vi "FPGA_HoppingScan.vi"() -> ()   [LabVIEW 2024]
uses:
  <vilib>/Platform/TimedLoop/XDataNode/timing_clust.ctl
  <vilib>/Platform/TimedLoop/XDataNode/nitl_modes.ctl
  <vilib>/Platform/TimedLoop/XDataNode/wakeup.ctl
  <vilib>/rvi/FXPMathLib/FxpDiv/subVIs/nifxpmath_Div_SimConfig.ctl
  <vilib>/rvi/Emulation/niFpgaSctlEmulationGetInTimedLoop.vi
  <vilib>/rvi/Emulation/niFpgaProcessEmulError.vi
  <vilib>/rvi/eio/common/nirviEmuTemplateMethod_errors.vi
  <vilib>/rvi/Emulation/niFpgaGetClockAttributes.vi
  <vilib>/rvi/Emulation/niFpgaEmulationReportErrorSimple.vi
  <vilib>/rvi/Emulation/niFpgaEmulationIsFPGAContextNoSignature.vi
  <vilib>/rvi/DataTransferAndStorage/Container/Common/niFpgaContainerGetUniqueNameForEmu.vi
  <vilib>/rvi/Memory/Memory_Emulation/niFpgaMemoryEmulationCacheClearOnFirstRun.vi
  <vilib>/rvi/Memory/Memory_Emulation/nirvimemoryEmulationManagerCache_MakeExclusive.vi
  <vilib>/rvi/Memory/Memory_Emulation/niFpgaMemoryEmulationValidateCache.vi
  <vilib>/rvi/Memory/Memory_Emulation/nirvimemoryEmulationManagerCache_InsertValue.vi
  <vilib>/Utility/error.llb/Clear Errors.vi
  <vilib>/rvi/Memory/Memory_Emulation/nirvimemoryEmulationManagerCache_ReleaseExclusive.vi
  <vilib>/rvi/Memory/Memory_Emulation/nirvimemoryEmulationManagerCache_GetValue.vi
  <vilib>/rvi/Memory/Memory_Emulation/nirvimemoryEmulationManagerCache_SetValue.vi
  <vilib>/rvi/FIFO/Fifo_Resource/nirvififoEmulationSetSize.vi
  <vilib>/rvi/FIFO/Fifo_Resource/nirviFifoEmulationQueueMgr.vi
  <instcachedir>/0/nirviFifoEmulationQueueMgr_E5CAEC123FF24DC58D834DCA3CDAA9B5.lvgen/nirviFifoEmulationQueueMgr_E5CAEC123FF24DC58D834DCA3CDAA9B5_001.vi
  <vilib>/rvi/errors/niFpgaSetErrorForExecOnDevCompSimple.vi
  <vilib>/rvi/eio/common/nirviEmuReportErrorAndStop.vi
  <vilib>/rvi/FIFO/Fifo_Resource/nirvififoEmulationCreateLock.vi
  <vilib>/rvi/FIFO/Fifo_Resource/nirvififoEmulationObtainLock.vi
  <vilib>/rvi/FIFO/Fifo_Resource/nirvififoEmulationReleaseLock.vi
  <vilib>/rvi/occurrence/nirviWaitOnOccurrenceBase.vi
  <vilib>/rvi/errors/nirviReportUnexpectedCaseInternalError.vi
  <vilib>/rvi/errors/nirviReportUnexpectedCaseInternalError (U32).vi
  <vilib>/rvi/Emulation/niFpgaCriticalErrorInLSC.vi
  <vilib>/rvi/Memory/Memory_Emulation/nirvimemoryFastEmulation.vi
  <vilib>/rvi/Memory/Memory_Emulation/nirvimemoryEmulation.vi
  <vilib>/eio/utilities/niEioResolveVilibRelativePath.vi
  <vilib>/rvi/interface/RandomDataEmulation/niFpgaRandomDataHandleErrors.vi
  <vilib>/rvi/FXPMathLib/FxpDiv/simVIs/DllFxpDivTemp_sub.vi
  <vilib>/rvi/FIFO/Fifo_Resource/nirvififoEmulationDetermineInputValidOut.vi
  <vilib>/eio/EIONode/EIONode.xnode
  <vilib>/rvi/DataTransferAndStorage/Container/XNode/niFpgaContainer.xnode
  <vilib>/rvi/DataTransferAndStorage/Register/Emulation/niFpgaRegisterEmulation.vi
  <vilib>/rvi/FIFO/Fifo_Resource/nirvififoEmulationGetNumberOfElementsToRead.vi
  <vilib>/rvi/FIFO/Fifo_Resource/nirvififoEmulationRead.vi
  <vilib>/platform/TimedLoop/XDataNode/XDataNode.xnode
  <vilib>/rvi/interface/RandomDataEmulation/nirviRandomDataFpgaReadWriteTemplate.vi
  <vilib>/rvi/FXPMathLib/FxpSub/XNode/nifxpmath_Sub.xnode
  <vilib>/rvi/FXPMathLib/FxpAdd/XNode/nifxpmath_Add.xnode
  <vilib>/rvi/FXPMathLib/FxpMul/XNode/nifxpmath_Multiplier.xnode
  <vilib>/rvi/FXPMathLib/FxpDiv/XNode/nifxpmath_Div.xnode
  <vilib>/rvi/FIFO/Fifo_Resource/nirvififoEmulationWrite.vi
  <vilib>/rvi/FXPMathLib/sim/FxpSim.dll
  <vilib>/Platform/TimedLoop/XDataNode/XDNodeRunTimeDep.lvlib
panel:
  in  "DelayPoints":i32
  in  "Halting Threshold":fxp<+/-,48,16>
  out "point_scanned":u32
  in  "TotalPoints":u32
  in  "RetRate us":i32
  in  "AppRate_NF us":i32
  in  "AppRate_FF us":i32
  in  "Recording Threshold":fxp<+/-,48,16>
  in  "stop":bool
  out "TargetDone?":bool
  out "ScanFinished?":bool
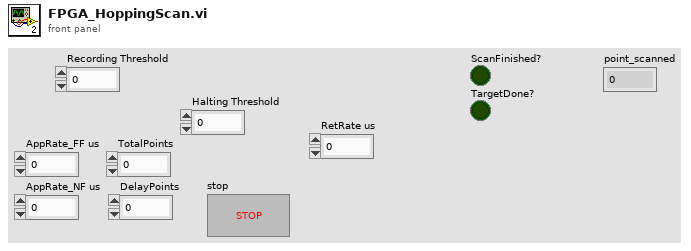
[diagram p1: front panel]
types:
  T1 = typedef "XDNodeRunTimeDep.lvlib/timing_clust.ctl" = cluster{"Expected End [f-1]":u64, "Actual End [f-1]":u64, "Finished Late? [f-1]":bool, "Expected End [i-1]":u64, "Actual End [i-1]":u64, "Finished Late? [i-1]":bool, "Expected Start [i]":u64, "Actual Start [i]":u64, "Expected Start [f]":u64, "Actual Start [f]":u64, "Source Name":string, "Structure Name":string, "Period":i64, "Deadline":i64, "Offset":i64, "Start":i64, "Priority":i32, "Timeout":i32, "Mode":T2, "Wakeup Reason":T3, "Error":errorcluster, "Source Type":string, "Secondary Source Type":string, "Global End Time":u64, "Global Start Time":u64, "Frame Duration":u64, "Iteration Duration":u64, "Assigned CPU":i32, "I/O Scan Engine Mode":u32}
  T2 = typedef "XDNodeRunTimeDep.lvlib/nitl_modes.ctl" = enum32{"No Change", "Process missed periods, maintain original phase", "Discard missed periods, maintain original phase", "Process missed periods, ignore original phase", "Discard missed periods, ignore original phase"}
  T3 = typedef "XDNodeRunTimeDep.lvlib/wakeup.ctl" = enum32{"Normal", "Aborted", "Asynchronous wakeup", "Timing source error", "Timed loop error", "Timeout"}
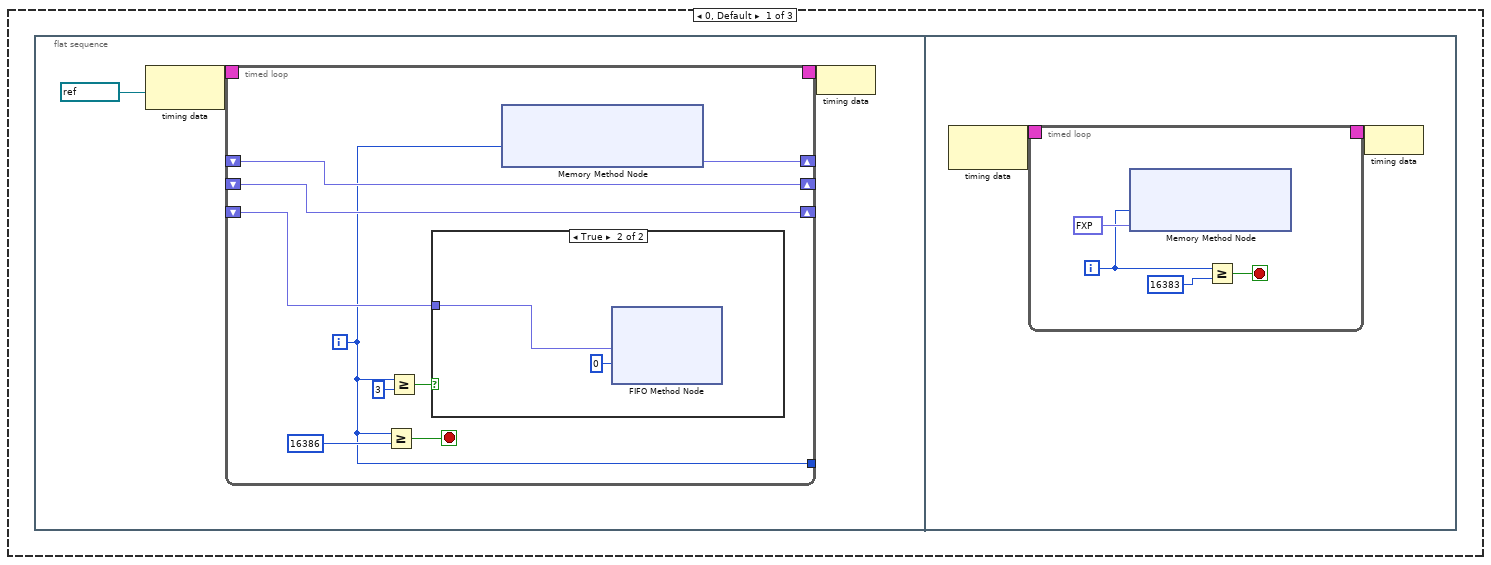
[diagram p3: hidden frame]
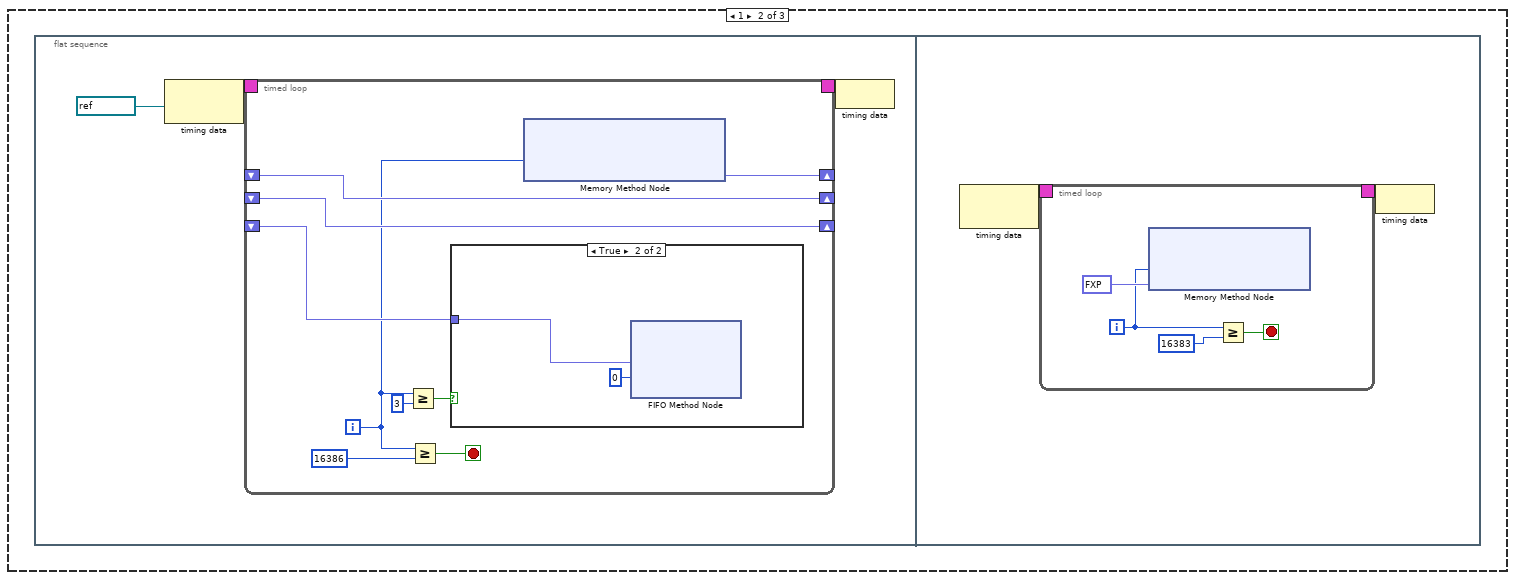
[diagram p5: hidden frame]
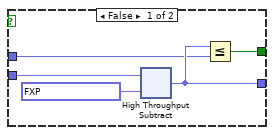
[diagram p13: hidden frame]
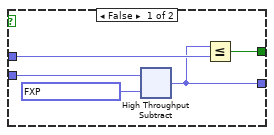
[diagram p14: hidden frame]
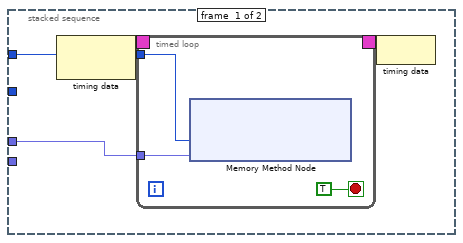
[diagram p16: hidden frame]
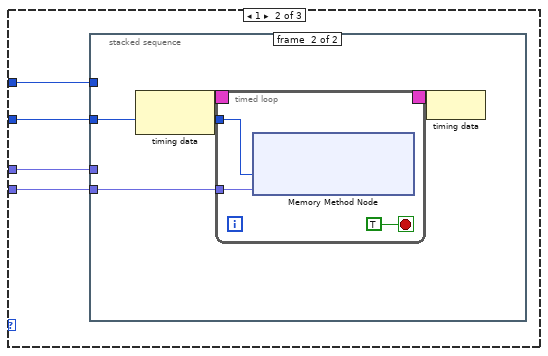
[diagram p17: hidden frame]
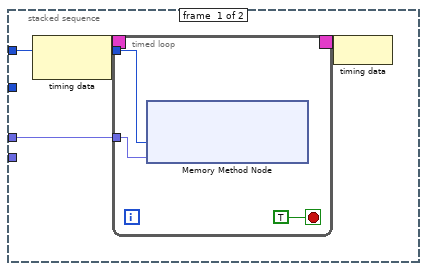
[diagram p18: hidden frame]
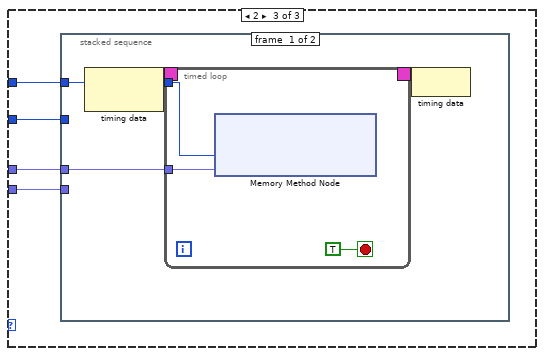
[diagram p19: hidden frame]
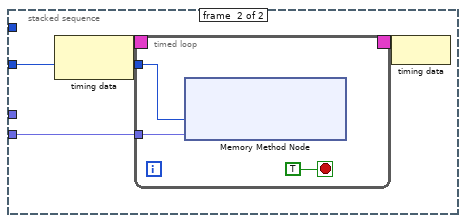
[diagram p20: hidden frame]
diagram:
  n1 = flat-sequence {
    tunnel: [w5] -> w1
    tunnel: w1 -> [w18]
    frame #0 {
      w4 = fxp<+/-,20,5> 0.0 ("Connector0/AO0")
      n2 = xnode "FPGA I/O Node"("Connector0/AO0"=w4, "Connector0/AO1"=w4, "Connector0/AO2"=w4) -> ()  [unwired: 3 in, 3 out]
      "ScanFinished?" <- FALSE
      "TargetDone?" <- FALSE
    }
    frame #1 {
      n3 = Generate Occurrence() -> (w5:refnum<k4>)
      n4 = call "Wait"("Count(mSec)"=u8 200) -> ()  [unwired: 1 out]
    }
    frame #2 {
      n5 = while {
        tunnel: w18 -> [w135]
        stop <- w137 stop-if-true
        n6 = xnode ("Register Read")() -> ("Data"=w138:bool)  [unwired: 1 in, 1 out]
        n7 = xnode ("FIFO Method Node")() -> ("Number of Elements to Read"=w141:u32)  [unwired: 1 in, 1 out]
        n8 = local read "ScanFinished?"() -> (w136:bool)
        n9 = Or(x=w138, y=w136) -> (x .or. y?=w137:bool)
        n10 = Greater Or Equal?(x=w141, y=u32 6) -> (x >= y?=w139:bool)
        n11 = case shown="True" w139 {
          tunnel: w135 -> [_ w142]
          frame False {
          }
          frame True {
            n12 = First Call?() -> (First Call?: T/F=w143:bool)
            n13 = case shown="True" w143 {
              tunnel: w142 -> [_ w144]
              frame False {
              }
              frame True {
                n14 = flat-sequence {
                  tunnel: [w147] -> w145
                  tunnel: w144 -> [w147]
                  tunnel: w145 -> [w148]
                  frame #0 {
                    n15 = call "Wait3"("Count(mSec)"=u8 4) -> ()  [unwired: 1 out]
                  }
                  frame #1 {
                    n16 = Set Occurrence(w148) -> ()
                  }
                }
              }
            }
          }
        }
      }
      n17 = while {
        tunnel: w18 -> [w120]
        stop <- w117 stop-if-true
        n18 = flat-sequence {
          tunnel: ["stop"] -> w122
          tunnel: w120 -> [w124]
          tunnel: [w124] -> w118
          tunnel: w122 -> [w127]
          tunnel: [w127] -> w121
          tunnel: [w126] -> w119
          tunnel: w118 -> [w126]
          tunnel: w121 -> [w131]
          tunnel: w119 -> [w130]
          tunnel: [w129] -> w117
          frame #0 {
            n19 = case shown="True" "stop" {
              tunnel: "stop" -> [_ w125]
              frame False {
              }
              frame True {
                n20 = xnode ("Register Write")("Data"=w125) -> ()  [unwired: 1 in, 1 out]
              }
            }
          }
          frame #1 {
            n21 = call "Wait2"("Count(uSec)"=u8 200) -> ()  [unwired: 1 out]
          }
          frame #2 {
            n22 = xnode ("Register Read")() -> ("Data"=w132:bool)  [unwired: 1 in, 1 out]
            n23 = local read "ScanFinished?"() -> (w133:bool)
            n24 = Compound Arithmetic op=OR(w133, w132, w131) -> (w129:bool)
            n25 = case shown="True" w129 {
              tunnel: w130 -> [_ w134]
              frame False {
              }
              frame True {
                n26 = Set Occurrence(w134) -> ()
              }
            }
          }
        }
      }
      n27 = flat-sequence {
        tunnel: w18 -> [w149]
        tunnel: [fxp<+/-,48,16> 0.0 ("Threshold")] -> w17
        tunnel: [w151] -> w15
        tunnel: [u8 0] -> w12
        tunnel: w17 -> [w154]
        tunnel: [w155] -> w16
        tunnel: w15 -> [w155]
        tunnel: [w154] -> w14
        tunnel: [w153] -> w13
        tunnel: w12 -> [w153]
        tunnel: w16 -> [w160]
        tunnel: w14 -> [w159]
        tunnel: w13 -> [w158]
        tunnel: [w157] -> w11
        tunnel: w11 -> [w1114]
        tunnel: [w1112] -> w10
        tunnel: [w1111] -> w8
        tunnel: w10 -> [w1126]
        tunnel: [w1126] -> w9
        tunnel: w8 -> [w1125]
        tunnel: [w1125] -> w7
        tunnel: w9 -> [w1130]
        tunnel: w7 -> [w1127]
        frame #0 {
          n28 = Wait on Occurrence(2:w149) -> ()  [unwired: 2 in, 1 out]
        }
        frame #1 {
          # "z piezo voltage"
          # "Swapchain indicator"
          n29 = xnode ("Register Read")() -> ("Data"=w151:bool)  [unwired: 1 in, 1 out]
        }
        frame #2 {
          n30 = call "Wait4"("Count(mSec)"=u8 4) -> ()  [unwired: 1 out]
        }
        frame #3 {
          n31 = case shown="False" w160 {
            tunnel: w159 -> [w163 w1110]
            tunnel: w158 -> [w162 _]
            tunnel: [w161 w1110] -> w157
            frame False {
              n32 = while {
                shift-right: [w171] -> w161
                shift-left: w163 -> [w205]
                shift-right: [w170] -> _
                shift-left: w162 -> [w184]
                stop <- w169 stop-if-true
                n33 = flat-sequence {
                  tunnel: w205 -> [w207]
                  tunnel: [w209] -> w204
                  tunnel: [w208] -> w200
                  tunnel: [w207] -> w189
                  tunnel: w184 -> [w206]
                  tunnel: [w206] -> w183
                  tunnel: w204 -> [w217]
                  tunnel: [w217] -> w203
                  tunnel: w200 -> [w216]
                  tunnel: [w216] -> w199
                  tunnel: w189 -> [w215]
                  tunnel: [w215] -> w188
                  tunnel: w183 -> [w214]
                  tunnel: [w214] -> w182
                  tunnel: w203 -> [w244]
                  tunnel: [w244] -> w202
                  tunnel: [w237] -> w201
                  tunnel: w199 -> [w243]
                  tunnel: [w243] -> w198
                  tunnel: [w238] -> w196
                  tunnel: [w241] -> w194
                  tunnel: [w240] -> w193
                  tunnel: [w239] -> w192
                  tunnel: w188 -> [w236]
                  tunnel: w182 -> [w242]
                  tunnel: [w242] -> w181
                  tunnel: [w233] -> w168
                  tunnel: [w235] -> w164
                  tunnel: w202 -> [w280]
                  tunnel: w201 -> [w281]
                  tunnel: w198 -> [w279]
                  tunnel: [w279] -> w197
                  tunnel: w196 -> [w278]
                  tunnel: [w278] -> w195
                  tunnel: w194 -> [w277]
                  tunnel: w193 -> [w275]
                  tunnel: w192 -> [w274]
                  tunnel: [w277] -> w191
                  tunnel: [w272] -> w187
                  tunnel: w181 -> [w276]
                  tunnel: [w276] -> w180
                  tunnel: [w275] -> w177
                  tunnel: [w274] -> w176
                  tunnel: w168 -> [w273]
                  tunnel: [w273] -> w167
                  tunnel: w164 -> [w272]
                  tunnel: w197 -> [w308]
                  tunnel: w195 -> [w309]
                  tunnel: w191 -> [w307]
                  tunnel: [w307] -> w190
                  tunnel: w187 -> [w306]
                  tunnel: [w306] -> w186
                  tunnel: w180 -> [w305]
                  tunnel: [w305] -> w178
                  tunnel: w177 -> [w304]
                  tunnel: w176 -> [w303]
                  tunnel: [w304] -> w175
                  tunnel: [w303] -> w174
                  tunnel: w167 -> [w302]
                  tunnel: [w302] -> w166
                  tunnel: w190 -> [w335]
                  tunnel: w186 -> [w334]
                  tunnel: [w334] -> w185
                  tunnel: [w333] -> w179
                  tunnel: w178 -> [w333]
                  tunnel: w175 -> [w332]
                  tunnel: w174 -> [w331]
                  tunnel: [w332] -> w173
                  tunnel: [w331] -> w172
                  tunnel: w166 -> [w330]
                  tunnel: [w330] -> w165
                  tunnel: w185 -> [w350]
                  tunnel: w179 -> [w349]
                  tunnel: w173 -> [w348]
                  tunnel: w172 -> [w347]
                  tunnel: [w346] -> w170
                  tunnel: [w345] -> w171
                  tunnel: [w344] -> w169
                  tunnel: w165 -> [w340]
                  frame #0 {
                    # "Data from target to host:\n0, 1: X, Y piezo voltage\n2, 3: X, Y piezo idx\n4: Z piezo voltage\n5: baseline current\n(6-8105): Z voltage\n(8106-16205): current"
                    # "Data from host to target:\n0, 1: X, Y piezo voltage\n2, 3: X, Y piezo idx\n4: distance (piezo voltage) to the last point\n5: retract height, \nall negative cases won't trigger approach of z piezo\nif -20, keep z and move xy\nif -30, full retract for z and move xy"
                    n34 = for {
                      N: 2 -> [_]
                      shift-right: [w213] -> w208
                      shift-left: _ -> [w211]
                      shift-right: [w211] -> w209
                      shift-left: _ -> [_]
                      i -> [w212]
                      n35 = xnode ("Memory Method Node")("Address"=w212) -> ("Data"=w213:fxp<+/-,48,16>)  [unwired: 1 in, 1 out]
                    }
                  }
                  frame #1 {
                    # "y"
                    # "x"
                    n36 = while {
                      shift-right: [w221] -> _
                      shift-left: i16 0 -> [w220]
                      stop <- w222 stop-if-true
                      n37 = xnode ("FIFO Method Node")("Timeout"=8192) -> ("Element"=w219:fxp<+/-,48,16>, "Timed Out?"=w226:bool)  [unwired: 1 in, 1 out]
                      n38 = Increment(x=w220) -> (x+1=w229:i16)
                      n39 = xnode ("Register Read")() -> ("Data"=w223:bool)  [unwired: 1 in, 1 out]
                      n40 = Select(t=w220, s=w226, f=w229) -> (s? t:f=w221:i16)
                      n41 = Not(x=w226) -> (.not. x?=w225:bool)
                      n42 = Equal?(x=w220, y=i16 5) -> (x = y?=w227:bool)
                      n43 = And(x=w227, y=w225) -> (x .and. y?=w224:bool)
                      n44 = xnode ("Memory Method Node")("Address"=w220, "Data"=w219) -> ()  [unwired: 1 in, 1 out]
                      n45 = Or(x=w224, y=w223) -> (x .or. y?=w222:bool)
                    }
                  }
                  frame #2 {
                    # "0"
                    # "5"
                    n46 = for {
                      N: 6 -> [_]
                      shift-right: [w270] -> w233
                      shift-left: _ -> [w269]
                      shift-right: [w269] -> w241
                      shift-left: _ -> [w268]
                      shift-right: [w268] -> w240
                      shift-left: _ -> [w267]
                      shift-right: [w267] -> w239
                      shift-left: _ -> [w266]
                      shift-right: [w266] -> w238
                      shift-left: _ -> [w265]
                      shift-right: [w265] -> w237
                      shift-left: _ -> [_]
                      i -> [w271]
                      n47 = xnode ("Memory Method Node")("Address"=w271) -> ("Data"=w270:fxp<+/-,48,16>)  [unwired: 1 in, 1 out]
                    }
                    n48 = Equal?(x=w233, y=fxp<+/-,48,16> -30.0) -> (x = y?=w232:bool)
                    n49 = case shown="True" w232 {
                      tunnel: w236 -> [w246 w250]
                      tunnel: [w246 w249] -> w235
                      tunnel: fxp<+/-,48,16> 0.0048828125 ("y") -> [_ w248]
                      frame False {
                      }
                      frame True {
                        n50 = flat-sequence {
                          tunnel: w250 -> [w253]
                          tunnel: w248 -> [w251]
                          tunnel: [w252] -> w247
                          tunnel: [w264] -> w249
                          tunnel: w247 -> [w264]
                          frame #0 {
                            n51 = while {
                              shift-right: [w257] -> w252
                              shift-left: w253 -> [w262]
                              tunnel: w251 -> [w256]
                              stop <- w258 stop-if-true
                              w259 = fxp<+/-,48,16> 0.0 ("y")
                              n52 = xnode "High Throughput Subtract"("x"=w262, "y"=w256) -> ("x-y"=w260:fxp<+/-,48,16>)
                              n53 = xnode ("Register Read")() -> ("Data"=w261:bool)  [unwired: 1 in, 1 out]
                              n54 = Less Or Equal?(x=w260, y=w259) -> (x <= y?=w254:bool)
                              n55 = Select(t=w259, s=w254, f=w260) -> (s? t:f=w257:fxp<+/-,48,16>)
                              n56 = local read "RetRate us"() -> (w255:i32)
                              n57 = xnode "FPGA I/O Node"("Connector0/AO2"=w257) -> ()  [unwired: 1 in, 1 out]
                              n58 = Compound Arithmetic op=OR(w254, w261) -> (w258:bool)
                              n59 = call "Wait10"("Count(uSec)"=w255) -> ()  [unwired: 1 out]
                            }
                          }
                          frame #1 {
                            n60 = call "Wait17"("Count(mSec)"=u16 2 ("Count(uSec)")) -> ()  [unwired: 1 out]
                          }
                        }
                      }
                    }
                  }
                  frame #3 {
                    n61 = xnode "High Throughput Subtract"("x"=w280, "y"=w281) -> ("x-y"=w283:fxp<+/-,48,16>)
                    n62 = Less Or Equal To 0?(x=w283) -> (x <= 0?=w282:bool)
                    n63 = while {
                      tunnel: w282 -> [w291]
                      tunnel: w281 -> [w290]
                      shift-right: [w284] -> _
                      shift-left: w280 -> [w286]
                      stop <- w287 stop-if-true
                      n64 = case shown="True" w291 {
                        tunnel: w290 -> [w292 w297]
                        tunnel: w286 -> [w295 w301]
                        tunnel: [w294 w299] -> w285
                        tunnel: [w293 w298] -> w284
                        frame False {
                          n65 = xnode "High Throughput Subtract"("x"=w295, "y"=fxp<+/-,48,16> 0.00030517578125) -> ("x-y"=w293:fxp<+/-,48,16>)
                          n66 = Less Or Equal?(x=w293, y=w292) -> (x <= y?=w294:bool)
                        }
                        frame True {
                          n67 = xnode ("High Throughput Add")("x"=w301, "y"=fxp<+/-,48,16> 0.00030517578125) -> ("x+y"=w298:fxp<+/-,48,16>)
                          n68 = Greater Or Equal?(x=w298, y=w297) -> (x >= y?=w299:bool)
                        }
                      }
                      n69 = call "Wait5"("Count(uSec)"=u32 70) -> ()  [unwired: 1 out]
                      n70 = xnode ("Register Read")() -> ("Data"=w288:bool)  [unwired: 1 in, 1 out]
                      n71 = xnode "FPGA I/O Node"("Connector0/AO0"=w284) -> ()  [unwired: 1 in, 1 out]
                      n72 = Or(x=w285, y=w288) -> (x .or. y?=w287:bool)
                    }
                  }
                  frame #4 {
                    n73 = xnode "High Throughput Subtract"("x"=w308, "y"=w309) -> ("x-y"=w311:fxp<+/-,48,16>)
                    n74 = Less Or Equal To 0?(x=w311) -> (x <= 0?=w310:bool)
                    n75 = while {
                      tunnel: w310 -> [w319]
                      tunnel: w309 -> [w318]
                      shift-right: [w312] -> _
                      shift-left: w308 -> [w314]
                      stop <- w315 stop-if-true
                      n76 = case shown="True" w319 {
                        tunnel: w318 -> [w321 w326]
                        tunnel: w314 -> [w323 w329]
                        tunnel: [w322 w327] -> w313
                        tunnel: [w320 w325] -> w312
                        frame False {
                          n77 = xnode "High Throughput Subtract"("x"=w323, "y"=fxp<+/-,48,16> 0.00030517578125) -> ("x-y"=w320:fxp<+/-,48,16>)
                          n78 = Less Or Equal?(x=w320, y=w321) -> (x <= y?=w322:bool)
                        }
                        frame True {
                          n79 = xnode ("High Throughput Add")("x"=w329, "y"=fxp<+/-,48,16> 0.00030517578125) -> ("x+y"=w325:fxp<+/-,48,16>)
                          n80 = Greater Or Equal?(x=w325, y=w326) -> (x >= y?=w327:bool)
                        }
                      }
                      n81 = call "Wait6"("Count(uSec)"=u32 70) -> ()  [unwired: 1 out]
                      n82 = xnode ("Register Read")() -> ("Data"=w316:bool)  [unwired: 1 in, 1 out]
                      n83 = xnode "FPGA I/O Node"("Connector0/AO1"=w312) -> ()  [unwired: 1 in, 1 out]
                      n84 = Or(x=w313, y=w316) -> (x .or. y?=w315:bool)
                    }
                  }
                  frame #5 {
                    n85 = xnode ("High Throughput Multiply")("x"=w335, "y"=fxp<+/-,48,16> 1600.0) -> ("x*y"=w337:fxp<+/-,52,20>)
                    n86 = To Unsigned Long Integer(number=w337) -> (unsigned 32bit integer=w338:u32)
                    n87 = call "Wait7"("Count(uSec)"=w338) -> ()  [unwired: 1 out]
                  }
                  frame #6 {
                    # "Y, X idx"
                    n88 = xnode ("Register Read")() -> ("Data"=w343:bool)  [unwired: 1 in, 1 out]
                    n89 = Less Or Equal?(x=w340, y=fxp<+/-,48,16> -20.0) -> (x <= y?=w341:bool)
                    n90 = Or(x=w341, y=w343) -> (x .or. y?=w342:bool)
                    n91 = case shown="False" w342 {
                      tunnel: w350 -> [w370 w1109]
                      tunnel: w349 -> [w368 w1108]
                      tunnel: w348 -> [w362 _]
                      tunnel: w347 -> [w361 _]
                      tunnel: [w359 w1109] -> w345
                      tunnel: [w360 w1108] -> w346
                      tunnel: [w358 w1105] -> w344
                      tunnel: w341 -> [_ w1107]
                      tunnel: w340 -> [w354 _]
                      frame False {
                        n92 = flat-sequence {
                          tunnel: [w376] -> w373
                          tunnel: [w381] -> w372
                          tunnel: [w380] -> w371
                          tunnel: w370 -> [w379]
                          tunnel: [w379] -> w369
                          tunnel: w368 -> [w378]
                          tunnel: [w378] -> w367
                          tunnel: [0] -> w366
                          tunnel: [w376] -> w353
                          tunnel: [FALSE] -> w351
                          tunnel: w373 -> [w427]
                          tunnel: w372 -> [w426]
                          tunnel: w371 -> [w425]
                          tunnel: w369 -> [w424]
                          tunnel: w367 -> [w423]
                          tunnel: w366 -> [w418]
                          tunnel: [w422] -> w365
                          tunnel: [w421] -> w364
                          tunnel: [w420] -> w363
                          tunnel: w353 -> [w419]
                          tunnel: [w419] -> w352
                          tunnel: w351 -> [w417]
                          tunnel: w365 -> [w759]
                          tunnel: w364 -> [w761]
                          tunnel: w363 -> [w762]
                          tunnel: w362 -> [w764]
                          tunnel: w361 -> [w763]
                          tunnel: [w760] -> w357
                          tunnel: [w759] -> w356
                          tunnel: [w756] -> w355
                          tunnel: w352 -> [w755]
                          tunnel: [w1085] -> w358
                          tunnel: [w1084] -> w359
                          tunnel: [w1086] -> w360
                          tunnel: w357 -> [w1086]
                          tunnel: w356 -> [w1081]
                          tunnel: w355 -> [w1085]
                          tunnel: w354 -> [w1082]
                          frame #0 {
                            n93 = for {
                              N: 64 -> [_]
                              shift-right: [w414] -> w384
                              shift-left: fxp<+/-,48,16> 0.0 -> [w415]
                              n94 = xnode "FPGA I/O Node"() -> ("Connector0/AI3"=w416:fxp<+/-,27,5>)  [unwired: 1 in, 1 out]
                              n95 = xnode ("High Throughput Add")("x"=w416, "y"=w415) -> ("x+y"=w414:fxp<+/-,48,16>)
                            }
                            n96 = local read "Halting Threshold"() -> (w375:fxp<+/-,48,16>)
                            n97 = local read "Recording Threshold"() -> (w382:fxp<+/-,48,16>)
                            n98 = xnode "High Throughput Divide"("x"=w384, "y"=fxp<+/-,48,16> 64.0) -> ("x/y"=w376:fxp<+/-,48,16>)
                            n99 = xnode ("High Throughput Multiply")("x"=w376, "y"=w382) -> ("x*y"=w381:fxp<+/-,48,16>)
                            n100 = xnode ("High Throughput Multiply")("x"=w376, "y"=w375) -> ("x*y"=w380:fxp<+/-,48,16>)
                          }
                          frame #1 {
                            n101 = while {
                              tunnel: w427 -> [w492]
                              tunnel: w426 -> [w491]
                              tunnel: w425 -> [w490]
                              shift-right: [w469] -> w422
                              shift-left: w424 -> [w489]
                              shift-right: [w468] -> w421
                              shift-left: w423 -> [w488]
                              shift-right: [w449] -> _
                              shift-left: w418 -> [w487]
                              shift-right: [w450] -> _
                              shift-left: w418 -> [w476]
                              tunnel: [w460] -> w420
                              shift-right: [w434] -> _
                              shift-left: w418 -> [w438]
                              shift-right: [w428] -> _
                              shift-left: w417 -> [w432]
                              stop <- w465 stop-if-true
                              n102 = flat-sequence {
                                tunnel: w476 -> [w496]
                                tunnel: w487 -> [w497]
                                tunnel: w488 -> [w498]
                                tunnel: w489 -> [w499]
                                tunnel: w490 -> [w500]
                                tunnel: w491 -> [w501]
                                tunnel: w492 -> [w502]
                                tunnel: [w502] -> w459
                                tunnel: [w501] -> w458
                                tunnel: [w500] -> w457
                                tunnel: [w499] -> w456
                                tunnel: [w498] -> w455
                                tunnel: [w497] -> w454
                                tunnel: [w496] -> w453
                                tunnel: [w495] -> w452
                                tunnel: [w494] -> w439
                                tunnel: w438 -> [w494]
                                tunnel: [w493] -> w433
                                tunnel: w432 -> [w493]
                                tunnel: [w550] -> w486
                                tunnel: [w546] -> w485
                                tunnel: [w545] -> w484
                                tunnel: [w533] -> w480
                                tunnel: [w530] -> w479
                                tunnel: [w544] -> w475
                                tunnel: [w543] -> w473
                                tunnel: [w542] -> w470
                                tunnel: [w523] -> w467
                                tunnel: [w504] -> w463
                                tunnel: [w535] -> w461
                                tunnel: w459 -> [w557]
                                tunnel: w458 -> [w555]
                                tunnel: w457 -> [w525]
                                tunnel: w456 -> [w547]
                                tunnel: w455 -> [w543]
                                tunnel: w454 -> [w520]
                                tunnel: w453 -> [w544]
                                tunnel: w452 -> [w529]
                                tunnel: [w529] -> w451
                                tunnel: w439 -> [w509]
                                tunnel: [w510] -> w436
                                tunnel: w433 -> [w506]
                                tunnel: [w504] -> w431
                                tunnel: w486 -> [w630]
                                tunnel: w485 -> [w629]
                                tunnel: w484 -> [w631]
                                tunnel: [w631] -> w483
                                tunnel: [w630] -> w482
                                tunnel: [w629] -> w481
                                tunnel: w480 -> [w628]
                                tunnel: w479 -> [w627]
                                tunnel: [w628] -> w478
                                tunnel: [w627] -> w477
                                tunnel: w475 -> [w626]
                                tunnel: [w626] -> w474
                                tunnel: w473 -> [w625]
                                tunnel: [w625] -> w472
                                tunnel: [w624] -> w471
                                tunnel: w470 -> [w624]
                                tunnel: w467 -> [w623]
                                tunnel: [w623] -> w466
                                tunnel: [w622] -> w464
                                tunnel: w463 -> [w622]
                                tunnel: [w621] -> w462
                                tunnel: w461 -> [w621]
                                tunnel: w451 -> [w620]
                                tunnel: [w620] -> w442
                                tunnel: [w619] -> w437
                                tunnel: w436 -> [w619]
                                tunnel: w431 -> [w618]
                                tunnel: [w618] -> w430
                                tunnel: w483 -> [w638]
                                tunnel: w482 -> [w652]
                                tunnel: w481 -> [w643]
                                tunnel: w478 -> [w645]
                                tunnel: w477 -> [w644]
                                tunnel: w474 -> [w646]
                                tunnel: w472 -> [w642]
                                tunnel: w471 -> [w648]
                                tunnel: w466 -> [w641]
                                tunnel: w464 -> [w640]
                                tunnel: w462 -> [w639]
                                tunnel: [w652] -> w448
                                tunnel: [w647] -> w447
                                tunnel: [w643] -> w446
                                tunnel: [w642] -> w445
                                tunnel: [w641] -> w444
                                tunnel: [w639] -> w443
                                tunnel: w442 -> [w636]
                                tunnel: [w636] -> w441
                                tunnel: [w635] -> w440
                                tunnel: w437 -> [w633]
                                tunnel: [w633] -> w435
                                tunnel: w430 -> [w632]
                                tunnel: [w632] -> w429
                                tunnel: [w749] -> w460
                                tunnel: [w750] -> w465
                                tunnel: [w751] -> w468
                                tunnel: [w752] -> w469
                                tunnel: [w753] -> w450
                                tunnel: [w754] -> w449
                                tunnel: w448 -> [w754]
                                tunnel: w447 -> [w753]
                                tunnel: w446 -> [w752]
                                tunnel: w445 -> [w751]
                                tunnel: w444 -> [w750]
                                tunnel: w443 -> [w749]
                                tunnel: w441 -> [w747]
                                tunnel: w440 -> [w746]
                                tunnel: [w740] -> w434
                                tunnel: w435 -> [w740]
                                tunnel: w429 -> [w739]
                                tunnel: [w739] -> w428
                                frame #0 {
                                n103 = call "Tick Count"() -> ("Tick Count(uSec)"=w495:u32)
                                }
                                frame #1 {
                                w507 = 16
                                w522 = 1 ("y")
                                w548 = fxp<+/-,48,16> 0.0 ("y")
                                # "brake zone"
                                # "recording zone"
                                # "speed switch"
                                n104 = for {
                                N: w507 -> [_]
                                shift-right: [w615] -> w534
                                shift-left: w548 -> [w616]
                                shift-right: [w612] -> w532
                                shift-left: w548 -> [w614]
                                n105 = xnode "FPGA I/O Node"() -> ("Connector0/AI2"=w617:fxp<+/-,27,5>, "Connector0/AI3"=w613:fxp<+/-,27,5>)  [unwired: 2 in, 2 out]
                                n106 = xnode ("High Throughput Add")("x"=w614, "y"=w613) -> ("x+y"=w612:fxp<+/-,48,16>)
                                n107 = xnode ("High Throughput Add")("x"=w617, "y"=w616) -> ("x+y"=w615:fxp<+/-,48,16>)
                                }
                                n108 = To Fixed-Point(number=w507) -> (fixed-point=w531:fxp<+/-,48,16>)  [unwired: 1 in]
                                n109 = local read "DelayPoints"() -> (w503:i32)
                                n110 = Not Equal To 0?(x=w509) -> (x != 0?=w508:bool)
                                n111 = Greater Or Equal?(x=w509, y=w503) -> (x >= y?=w516:bool)
                                n112 = Select(t=fxp<+/-,48,16> 0.0 ("y"), s=w508, f=fxp<+/-,48,16> 0.00030517578125 ("y")) -> (s? t:f=w517:fxp<+/-,48,16>)
                                n113 = xnode "High Throughput Divide"("x"=w534, "y"=w531) -> ("x/y"=w533:fxp<+/-,48,16>)
                                n114 = xnode "High Throughput Divide"("x"=w532, "y"=w531) -> ("x/y"=w530:fxp<+/-,48,16>)
                                n115 = xnode ("High Throughput Add")("x"=w517, "y"=w547) -> ("x+y"=w536:fxp<+/-,48,16>)
                                n116 = xnode "High Throughput Subtract"("x"=w557, "y"=w530) -> ("x-y"=w556:fxp<+/-,48,16>)
                                n117 = Absolute Value(x=w556) -> (abs(x)=w526:fxp<+,48,16>)
                                n118 = Less Or Equal?(x=w536, y=fxp<+/-,48,16> 9.75) -> (x <= y?=w538:bool)
                                n119 = Greater Or Equal?(x=w536, y=fxp<+/-,48,16> -0.125) -> (x >= y?=w539:bool)
                                n120 = And(x=w539, y=w538) -> (x .and. y?=w537:bool)
                                n121 = Greater Or Equal?(x=w526, y=w555) -> (x >= y?=w554:bool)
                                n122 = Less Or Equal?(x=w526, y=w525) -> (x <= y?=w528:bool)
                                n123 = Increment(x=w520) -> (x+1=w553:i32)
                                n124 = Select(t=w553, s=w554, f=0) -> (s? t:f=w550:i32)
                                n125 = xnode ("Register Read")() -> ("Data"=w542:bool)  [unwired: 1 in, 1 out]
                                n126 = Greater Or Equal?(x=w550, y=w522) -> (x >= y?=w505:bool)
                                n127 = Equal?(x=w550, y=0 ("f")) -> (x = y?=w549:bool)
                                n128 = Not(x=w528) -> (.not. x?=w535:bool)
                                n129 = Or(x=w506, y=w505) -> (x .or. y?=w504:bool)
                                n130 = Select(t=1 ("y"), s=w504, f=0) -> (s? t:f=w512:i32)
                                n131 = Add(x=w509, y=w512) -> (x+y=w511:i32)
                                n132 = Select(t=0, s=w516, f=w511) -> (s? t:f=w510:i32)
                                n133 = Greater Or Equal?(x=w550, y=w522) -> (x >= y?=w545:bool)
                                n134 = Compound Arithmetic op=AND(w528, invert w542, w537) -> (w524:bool)
                                n135 = Or(x=w549, y=w504) -> (x .or. y?=w521:bool)
                                n136 = And(x=w521, y=w524) -> (x .and. y?=w527:bool)
                                n137 = Not(x=w524) -> (.not. x?=w523:bool)
                                n138 = Select(t=w536, s=w527, f=w547) -> (s? t:f=w546:fxp<+/-,48,16>)
                                }
                                frame #2 {
                                n139 = xnode "FPGA I/O Node"("Connector0/AO2"=w629) -> ()  [unwired: 1 in, 1 out]
                                }
                                frame #3 {
                                n140 = Compound Arithmetic op=AND(w640, invert w648) -> (w634:bool)
                                n141 = case shown="True" w634 {
                                tunnel: w642 -> [_ w660]
                                tunnel: w646 -> [_ w656]
                                tunnel: w645 -> [_ w654]
                                tunnel: w644 -> [_ w653]
                                frame False {
                                }
                                frame True {
                                n142 = Add(x=w656, y=6) -> (x+y=w658:i32)
                                n143 = Add(x=w656, y=8106) -> (x+y=w655:i32)
                                n144 = case shown="0, Default" w660 {
                                tunnel: w658 -> [w664 w688 w716]
                                tunnel: w655 -> [w663 w687 w715]
                                tunnel: w654 -> [w662 w689 w714]
                                tunnel: w653 -> [w661 w690 w713]
                                frame 0, Default {
                                n145 = stacked-sequence {
                                tunnel: w664 -> [w668 _]
                                tunnel: w663 -> [_ w679]
                                tunnel: w662 -> [w667 _]
                                tunnel: w661 -> [_ w678]
                                frame #0 {
                                n146 = node-c288() -> (w666:T1)  [unwired: 1 in]
                                n147 = timed-loop {
                                timing: w666 -> [_]
                                timing-out: [_] -> w665
                                tunnel: w668 -> [w671]
                                tunnel: w667 -> [w670]
                                stop <- TRUE stop-if-true
                                n148 = xnode ("Memory Method Node")("Address"=w671, "Data"=w670) -> ()  [unwired: 1 in, 1 out]
                                }
                                n149 = node-c288(w665) -> ()
                                }
                                frame #1 {
                                n150 = node-c288() -> (w677:T1)  [unwired: 1 in]
                                n151 = timed-loop {
                                timing: w677 -> [_]
                                timing-out: [_] -> w676
                                tunnel: w679 -> [w682]
                                tunnel: w678 -> [w681]
                                stop <- TRUE stop-if-true
                                n152 = xnode ("Memory Method Node")("Address"=w682, "Data"=w681) -> ()  [unwired: 1 in, 1 out]
                                }
                                n153 = node-c288(w676) -> ()
                                }
                                }
                                }
                                frame 1 {
                                n154 = stacked-sequence {
                                tunnel: w690 -> [_ w705]
                                tunnel: w689 -> [w694 _]
                                tunnel: w688 -> [w693 _]
                                tunnel: w687 -> [_ w704]
                                frame #0 {
                                n155 = node-c288() -> (w692:T1)  [unwired: 1 in]
                                n156 = timed-loop {
                                timing: w692 -> [_]
                                timing-out: [_] -> w691
                                tunnel: w694 -> [w697]
                                tunnel: w693 -> [w696]
                                stop <- TRUE stop-if-true
                                n157 = xnode ("Memory Method Node")("Address"=w696, "Data"=w697) -> ()  [unwired: 1 in, 1 out]
                                }
                                n158 = node-c288(w691) -> ()
                                }
                                frame #1 {
                                n159 = node-c288() -> (w703:T1)  [unwired: 1 in]
                                n160 = timed-loop {
                                timing: w703 -> [_]
                                timing-out: [_] -> w702
                                tunnel: w705 -> [w708]
                                tunnel: w704 -> [w707]
                                stop <- TRUE stop-if-true
                                n161 = xnode ("Memory Method Node")("Address"=w707, "Data"=w708) -> ()  [unwired: 1 in, 1 out]
                                }
                                n162 = node-c288(w702) -> ()
                                }
                                }
                                }
                                frame 2 {
                                n163 = stacked-sequence {
                                tunnel: w713 -> [_ w731]
                                tunnel: w714 -> [w720 _]
                                tunnel: w716 -> [w719 _]
                                tunnel: w715 -> [_ w730]
                                frame #0 {
                                n164 = node-c288() -> (w718:T1)  [unwired: 1 in]
                                n165 = timed-loop {
                                timing: w718 -> [_]
                                timing-out: [_] -> w717
                                tunnel: w720 -> [w721]
                                tunnel: w719 -> [w722]
                                stop <- TRUE stop-if-true
                                n166 = xnode ("Memory Method Node")("Address"=w722, "Data"=w721) -> ()  [unwired: 1 in, 1 out]
                                }
                                n167 = node-c288(w717) -> ()
                                }
                                frame #1 {
                                n168 = node-c288() -> (w729:T1)  [unwired: 1 in]
                                n169 = timed-loop {
                                timing: w729 -> [_]
                                timing-out: [_] -> w728
                                tunnel: w731 -> [w732]
                                tunnel: w730 -> [w733]
                                stop <- TRUE stop-if-true
                                n170 = xnode ("Memory Method Node")("Address"=w733, "Data"=w732) -> ()  [unwired: 1 in, 1 out]
                                }
                                n171 = node-c288(w728) -> ()
                                }
                                }
                                }
                                }
                                }
                                }
                                n172 = local read "AppRate_NF us"() -> (w651:i32)
                                n173 = local read "AppRate_FF us"() -> (w650:i32)
                                n174 = Increment(x=w646) -> (x+1=w649:i32)
                                n175 = Select(t=w651, s=w638, f=w650) -> (s? t:f=w635:i32)
                                n176 = Select(t=w649, s=w634, f=0) -> (s? t:f=w647:i32)
                                }
                                frame #4 {
                                n177 = call "Tick Count2"() -> ("Tick Count(uSec)"=w748:u32)
                                n178 = Subtract(x=w748, y=w747) -> (x-y=w745:i32)
                                n179 = Subtract(x=w746, y=w745) -> (x-y=w744:i32)
                                n180 = In Range and Coerce(upper limit=40000, x=w744, lower limit=1) -> (coerced(x)=w741:i32)  [unwired: 1 out]
                                n181 = call "Wait9"("Count(uSec)"=w741) -> ()  [unwired: 1 out]
                                }
                              }
                            }
                          }
                          frame #2 {
                            n182 = xnode ("Register Read")() -> ("Data"=w758:bool)  [unwired: 1 in, 1 out]
                            n183 = Compound Arithmetic op=AND(w762, invert w758) -> (w765:bool)
                            n184 = case shown="True" w765 {
                              tunnel: w764 -> [_ w785]
                              tunnel: w763 -> [_ w786]
                              tunnel: w761 -> [w767 w784]
                              tunnel: [w767 w783] -> w760
                              tunnel: [FALSE w779] -> w757
                              tunnel: w755 -> [_ w778]
                              frame False {
                              }
                              frame True {
                                w787 = fxp<+/-,48,16> 0.0 ("ZPeizoOffset")
                                n185 = for {
                                N: 16 -> [_]
                                shift-right: [w1073] -> w776
                                shift-left: w787 -> [w1077]
                                shift-right: [w1072] -> w773
                                shift-left: w787 -> [w1075]
                                shift-right: [w1069] -> w770
                                shift-left: w787 -> [w1071]
                                n186 = xnode "FPGA I/O Node"() -> ("Connector0/AI0"=w1076:fxp<+/-,27,5>, "Connector0/AI1"=w1074:fxp<+/-,27,5>, "Connector0/AI2"=w1070:fxp<+/-,27,5>)  [unwired: 3 in, 3 out]
                                n187 = xnode ("High Throughput Add")("x"=w1076, "y"=w1077) -> ("x+y"=w1073:fxp<+/-,48,16>)
                                n188 = xnode ("High Throughput Add")("x"=w1071, "y"=w1070) -> ("x+y"=w1069:fxp<+/-,48,16>)
                                n189 = xnode ("High Throughput Add")("x"=w1074, "y"=w1075) -> ("x+y"=w1072:fxp<+/-,48,16>)
                                }
                                n190 = feedback #1(u32 0 ("Timeout")) -> (w781:u32)
                                n191 = Increment(x=w781) -> (x+1=w768:u32)
                                "point_scanned" <- w768
                                n192 = feedback-in #1(w768) -> ()
                                n193 = local read "TotalPoints"() -> (w780:u32)
                                n194 = Greater Or Equal?(x=w768, y=w780) -> (x >= y?=w779:bool)
                                n195 = xnode "High Throughput Divide"("x"=w773, "y"=fxp<+/-,48,16> 16.0 ("ZPeizoOffset")) -> ("x/y"=w772:fxp<+/-,48,16>)
                                n196 = xnode "High Throughput Divide"("x"=w776, "y"=fxp<+/-,48,16> 16.0 ("ZPeizoOffset")) -> ("x/y"=w775:fxp<+/-,48,16>)
                                n197 = xnode "High Throughput Divide"("x"=w770, "y"=fxp<+/-,48,16> 16.0 ("ZPeizoOffset")) -> ("x/y"=w769:fxp<+/-,48,16>)
                                n198 = stacked-sequence {
                                tunnel: w775 -> [w870 _ _ _ _ _ _]
                                tunnel: w772 -> [_ w902 _ _ _ _ _]
                                tunnel: w769 -> [_ _ _ _ w998 _ _]
                                tunnel: w786 -> [_ _ w935 _ _ _ _]
                                tunnel: w785 -> [_ _ _ w967 _ _ _]
                                tunnel: w784 -> [w871 w903 w934 w966 w999 w1031 w1066]
                                tunnel: [_ _ _ _ _ _ w1064] -> w783
                                tunnel: w778 -> [_ _ _ _ _ w1030 _]
                                frame #0 {
                                n199 = case shown="2" w871 {
                                tunnel: w870 -> [w874 w884 w892]
                                frame 0, Default {
                                n200 = node-c288() -> (w873:T1)  [unwired: 1 in]
                                n201 = timed-loop {
                                timing: w873 -> [_]
                                timing-out: [_] -> w872
                                tunnel: w874 -> [w876]
                                stop <- TRUE stop-if-true
                                n202 = xnode ("Memory Method Node")("Address"=u32 0, "Data"=w876) -> ()  [unwired: 1 in, 1 out]
                                }
                                n203 = node-c288(w872) -> ()
                                }
                                frame 1 {
                                n204 = node-c288() -> (w883:T1)  [unwired: 1 in]
                                n205 = timed-loop {
                                timing: w883 -> [_]
                                timing-out: [_] -> w882
                                tunnel: w884 -> [w886]
                                stop <- TRUE stop-if-true
                                n206 = xnode ("Memory Method Node")("Address"=u32 0, "Data"=w886) -> ()  [unwired: 1 in, 1 out]
                                }
                                n207 = node-c288(w882) -> ()
                                }
                                frame 2 {
                                n208 = node-c288() -> (w894:T1)  [unwired: 1 in]
                                n209 = timed-loop {
                                timing: w894 -> [_]
                                timing-out: [_] -> w893
                                tunnel: w892 -> [w895]
                                stop <- TRUE stop-if-true
                                n210 = xnode ("Memory Method Node")("Address"=u32 0, "Data"=w895) -> ()  [unwired: 1 in, 1 out]
                                }
                                n211 = node-c288(w893) -> ()
                                }
                                }
                                }
                                frame #1 {
                                n212 = case shown="2" w903 {
                                tunnel: w902 -> [w906 w916 w924]
                                frame 0, Default {
                                n213 = node-c288() -> (w905:T1)  [unwired: 1 in]
                                n214 = timed-loop {
                                timing: w905 -> [_]
                                timing-out: [_] -> w904
                                tunnel: w906 -> [w908]
                                stop <- TRUE stop-if-true
                                n215 = xnode ("Memory Method Node")("Address"=u32 1, "Data"=w908) -> ()  [unwired: 1 in, 1 out]
                                }
                                n216 = node-c288(w904) -> ()
                                }
                                frame 1 {
                                n217 = node-c288() -> (w915:T1)  [unwired: 1 in]
                                n218 = timed-loop {
                                timing: w915 -> [_]
                                timing-out: [_] -> w914
                                tunnel: w916 -> [w918]
                                stop <- TRUE stop-if-true
                                n219 = xnode ("Memory Method Node")("Address"=u32 1, "Data"=w918) -> ()  [unwired: 1 in, 1 out]
                                }
                                n220 = node-c288(w914) -> ()
                                }
                                frame 2 {
                                n221 = node-c288() -> (w926:T1)  [unwired: 1 in]
                                n222 = timed-loop {
                                timing: w926 -> [_]
                                timing-out: [_] -> w925
                                tunnel: w924 -> [w927]
                                stop <- TRUE stop-if-true
                                n223 = xnode ("Memory Method Node")("Address"=u32 0, "Data"=w927) -> ()  [unwired: 1 in, 1 out]
                                }
                                n224 = node-c288(w925) -> ()
                                }
                                }
                                }
                                frame #2 {
                                n225 = case shown="2" w934 {
                                tunnel: w935 -> [w938 w948 w956]
                                frame 0, Default {
                                n226 = node-c288() -> (w937:T1)  [unwired: 1 in]
                                n227 = timed-loop {
                                timing: w937 -> [_]
                                timing-out: [_] -> w936
                                tunnel: w938 -> [w940]
                                stop <- TRUE stop-if-true
                                n228 = xnode ("Memory Method Node")("Address"=u32 2, "Data"=w940) -> ()  [unwired: 1 in, 1 out]
                                }
                                n229 = node-c288(w936) -> ()
                                }
                                frame 1 {
                                n230 = node-c288() -> (w947:T1)  [unwired: 1 in]
                                n231 = timed-loop {
                                timing: w947 -> [_]
                                timing-out: [_] -> w946
                                tunnel: w948 -> [w950]
                                stop <- TRUE stop-if-true
                                n232 = xnode ("Memory Method Node")("Address"=u32 2, "Data"=w950) -> ()  [unwired: 1 in, 1 out]
                                }
                                n233 = node-c288(w946) -> ()
                                }
                                frame 2 {
                                n234 = node-c288() -> (w958:T1)  [unwired: 1 in]
                                n235 = timed-loop {
                                timing: w958 -> [_]
                                timing-out: [_] -> w957
                                tunnel: w956 -> [w959]
                                stop <- TRUE stop-if-true
                                n236 = xnode ("Memory Method Node")("Address"=u32 0, "Data"=w959) -> ()  [unwired: 1 in, 1 out]
                                }
                                n237 = node-c288(w957) -> ()
                                }
                                }
                                }
                                frame #3 {
                                n238 = case shown="2" w966 {
                                tunnel: w967 -> [w970 w980 w988]
                                frame 0, Default {
                                n239 = node-c288() -> (w969:T1)  [unwired: 1 in]
                                n240 = timed-loop {
                                timing: w969 -> [_]
                                timing-out: [_] -> w968
                                tunnel: w970 -> [w972]
                                stop <- TRUE stop-if-true
                                n241 = xnode ("Memory Method Node")("Address"=u32 3, "Data"=w972) -> ()  [unwired: 1 in, 1 out]
                                }
                                n242 = node-c288(w968) -> ()
                                }
                                frame 1 {
                                n243 = node-c288() -> (w979:T1)  [unwired: 1 in]
                                n244 = timed-loop {
                                timing: w979 -> [_]
                                timing-out: [_] -> w978
                                tunnel: w980 -> [w982]
                                stop <- TRUE stop-if-true
                                n245 = xnode ("Memory Method Node")("Address"=u32 3, "Data"=w982) -> ()  [unwired: 1 in, 1 out]
                                }
                                n246 = node-c288(w978) -> ()
                                }
                                frame 2 {
                                n247 = node-c288() -> (w990:T1)  [unwired: 1 in]
                                n248 = timed-loop {
                                timing: w990 -> [_]
                                timing-out: [_] -> w989
                                tunnel: w988 -> [w991]
                                stop <- TRUE stop-if-true
                                n249 = xnode ("Memory Method Node")("Address"=u32 0, "Data"=w991) -> ()  [unwired: 1 in, 1 out]
                                }
                                n250 = node-c288(w989) -> ()
                                }
                                }
                                }
                                frame #4 {
                                n251 = case shown="2" w999 {
                                tunnel: w998 -> [w1002 w1012 w1020]
                                frame 0, Default {
                                n252 = node-c288() -> (w1001:T1)  [unwired: 1 in]
                                n253 = timed-loop {
                                timing: w1001 -> [_]
                                timing-out: [_] -> w1000
                                tunnel: w1002 -> [w1004]
                                stop <- TRUE stop-if-true
                                n254 = xnode ("Memory Method Node")("Address"=u32 4, "Data"=w1004) -> ()  [unwired: 1 in, 1 out]
                                }
                                n255 = node-c288(w1000) -> ()
                                }
                                frame 1 {
                                n256 = node-c288() -> (w1011:T1)  [unwired: 1 in]
                                n257 = timed-loop {
                                timing: w1011 -> [_]
                                timing-out: [_] -> w1010
                                tunnel: w1012 -> [w1014]
                                stop <- TRUE stop-if-true
                                n258 = xnode ("Memory Method Node")("Address"=u32 4, "Data"=w1014) -> ()  [unwired: 1 in, 1 out]
                                }
                                n259 = node-c288(w1010) -> ()
                                }
                                frame 2 {
                                n260 = node-c288() -> (w1022:T1)  [unwired: 1 in]
                                n261 = timed-loop {
                                timing: w1022 -> [_]
                                timing-out: [_] -> w1021
                                tunnel: w1020 -> [w1023]
                                stop <- TRUE stop-if-true
                                n262 = xnode ("Memory Method Node")("Address"=u32 0, "Data"=w1023) -> ()  [unwired: 1 in, 1 out]
                                }
                                n263 = node-c288(w1021) -> ()
                                }
                                }
                                }
                                frame #5 {
                                n264 = case shown="2" w1031 {
                                tunnel: w1030 -> [w1034 w1044 w1052]
                                frame 0, Default {
                                n265 = node-c288() -> (w1033:T1)  [unwired: 1 in]
                                n266 = timed-loop {
                                timing: w1033 -> [_]
                                timing-out: [_] -> w1032
                                tunnel: w1034 -> [w1036]
                                stop <- TRUE stop-if-true
                                n267 = xnode ("Memory Method Node")("Address"=u32 5, "Data"=w1036) -> ()  [unwired: 1 in, 1 out]
                                }
                                n268 = node-c288(w1032) -> ()
                                }
                                frame 1 {
                                n269 = node-c288() -> (w1043:T1)  [unwired: 1 in]
                                n270 = timed-loop {
                                timing: w1043 -> [_]
                                timing-out: [_] -> w1042
                                tunnel: w1044 -> [w1046]
                                stop <- TRUE stop-if-true
                                n271 = xnode ("Memory Method Node")("Address"=u32 5, "Data"=w1046) -> ()  [unwired: 1 in, 1 out]
                                }
                                n272 = node-c288(w1042) -> ()
                                }
                                frame 2 {
                                n273 = node-c288() -> (w1054:T1)  [unwired: 1 in]
                                n274 = timed-loop {
                                timing: w1054 -> [_]
                                timing-out: [_] -> w1053
                                tunnel: w1052 -> [w1055]
                                stop <- TRUE stop-if-true
                                n275 = xnode ("Memory Method Node")("Address"=u32 0, "Data"=w1055) -> ()  [unwired: 1 in, 1 out]
                                }
                                n276 = node-c288(w1053) -> ()
                                }
                                }
                                }
                                frame #6 {
                                n277 = xnode ("FIFO Method Node")("Element"=w1066, "Timeout"=0) -> ()  [unwired: 1 in, 2 out]
                                n278 = Increment(x=w1066) -> (x+1=w1065:u8)
                                n279 = Greater Or Equal?(x=w1065, y=u8 3) -> (x >= y?=w1067:bool)
                                n280 = Select(t=w1066, s=w1067, f=u8 0) -> (s? t:f=w1064:u8)
                                }
                                }
                              }
                            }
                            n281 = Or(x=w758, y=w757) -> (x .or. y?=w756:bool)
                          }
                          frame #3 {
                            n282 = xnode ("Register Read")() -> ("Data"=w1080:bool)  [unwired: 1 in, 1 out]
                            n283 = Less Or Equal To 0?(x=w1081) -> (x <= 0?=w1079:bool)
                            n284 = Or(x=w1080, y=w1079) -> (x .or. y?=w1078:bool)
                            n285 = case shown="False" w1078 {
                              tunnel: w1081 -> [w1089 w1103]
                              tunnel: [w1091 w1103] -> w1084
                              tunnel: fxp<+/-,48,16> 0.0048828125 ("y") -> [w1090 _]
                              tunnel: w1082 -> [w1087 _]
                              frame False {
                                n286 = xnode "High Throughput Subtract"("x"=w1089, "y"=w1087) -> ("x-y"=w1088:fxp<+/-,48,16>)
                                n287 = while {
                                shift-right: [w1096] -> w1091
                                shift-left: w1089 -> [w1102]
                                tunnel: w1090 -> [w1095]
                                tunnel: w1088 -> [w1094]
                                stop <- w1097 stop-if-true
                                n288 = xnode "High Throughput Subtract"("x"=w1102, "y"=w1095) -> ("x-y"=w1098:fxp<+/-,48,16>)
                                n289 = xnode ("Register Read")() -> ("Data"=w1101:bool)  [unwired: 1 in, 1 out]
                                n290 = Less Or Equal To 0?(x=w1098) -> (x <= 0?=w1099:bool)
                                n291 = Less Or Equal?(x=w1098, y=w1094) -> (x <= y?=w1100:bool)
                                n292 = Select(t=fxp<+/-,48,16> 0.0, s=w1099, f=w1098) -> (s? t:f=w1096:fxp<+/-,48,16>)
                                n293 = local read "RetRate us"() -> (w1092:i32)
                                n294 = xnode "FPGA I/O Node"("Connector0/AO2"=w1096) -> ()  [unwired: 1 in, 1 out]
                                n295 = Compound Arithmetic op=OR(w1099, w1100, w1101) -> (w1097:bool)
                                n296 = call "Wait11"("Count(uSec)"=w1092) -> ()  [unwired: 1 out]
                                }
                              }
                              frame True {
                              }
                            }
                          }
                        }
                      }
                      frame True {
                        n297 = xnode ("Register Read")() -> ("Data"=w1104:bool)  [unwired: 1 in, 1 out]
                        n298 = Not(x=w1107) -> (.not. x?=w1106:bool)
                        n299 = Or(x=w1106, y=w1104) -> (x .or. y?=w1105:bool)
                      }
                    }
                  }
                }
              }
            }
            frame True {
            }
          }
        }
        frame #4 {
          n300 = while {
            shift-right: [w1118] -> _
            shift-left: w1114 -> [w1123]
            tunnel: fxp<+/-,48,16> 0.0048828125 ("y") -> [w1117]
            stop <- w1119 stop-if-true
            w1115 = fxp<+/-,48,16> 0.0 ("t")
            n301 = xnode "High Throughput Subtract"("x"=w1123, "y"=w1117) -> ("x-y"=w1120:fxp<+/-,48,16>)
            n302 = Less Or Equal To 0?(x=w1120) -> (x <= 0?=w1121:bool)
            n303 = Less Or Equal?(x=w1120, y=w1115) -> (x <= y?=w1122:bool)
            n304 = Select(t=w1115, s=w1121, f=w1120) -> (s? t:f=w1118:fxp<+/-,48,16>)
            n305 = local read "RetRate us"() -> (w1116:i32)
            n306 = xnode "FPGA I/O Node"("Connector0/AO2"=w1118) -> ()  [unwired: 1 in, 1 out]
            n307 = Compound Arithmetic op=OR(w1121, w1122) -> (w1119:bool)
            n308 = call "Wait12"("Count(uSec)"=w1116) -> ()  [unwired: 1 out]
          }
          n309 = xnode "FPGA I/O Node"() -> ("Connector0/AI0"=w1112:fxp<+/-,27,5>, "Connector0/AI1"=w1111:fxp<+/-,27,5>)  [unwired: 2 in, 2 out]
        }
        frame #5 {
          n310 = call "Wait15"("Count(uSec)"=u8 100) -> ()  [unwired: 1 out]
        }
        frame #6 {
          n311 = while {
            shift-right: [w1134] -> _
            shift-left: w1127 -> [w1139]
            tunnel: fxp<+/-,48,16> 0.0048828125 ("y") -> [w1133]
            stop <- w1135 stop-if-true
            w1132 = fxp<+/-,48,16> 0.0 ("t")
            n312 = xnode "High Throughput Subtract"("x"=w1139, "y"=w1133) -> ("x-y"=w1136:fxp<+/-,48,16>)
            n313 = Less Or Equal To 0?(x=w1136) -> (x <= 0?=w1137:bool)
            n314 = Less Or Equal?(x=w1136, y=w1132) -> (x <= y?=w1138:bool)
            n315 = Select(t=w1132, s=w1137, f=w1136) -> (s? t:f=w1134:fxp<+/-,48,16>)
            n316 = xnode "FPGA I/O Node"("Connector0/AO1"=w1134) -> ()  [unwired: 1 in, 1 out]
            n317 = Compound Arithmetic op=OR(w1137, w1138) -> (w1135:bool)
            n318 = call "Wait14"("Count(uSec)"=u16 100) -> ()  [unwired: 1 out]
          }
          n319 = while {
            shift-right: [w1143] -> _
            shift-left: w1130 -> [w1148]
            tunnel: fxp<+/-,48,16> 0.0048828125 ("y") -> [w1142]
            stop <- w1144 stop-if-true
            w1141 = fxp<+/-,48,16> 0.0 ("t")
            n320 = xnode "High Throughput Subtract"("x"=w1148, "y"=w1142) -> ("x-y"=w1145:fxp<+/-,48,16>)
            n321 = Less Or Equal To 0?(x=w1145) -> (x <= 0?=w1146:bool)
            n322 = Less Or Equal?(x=w1145, y=w1141) -> (x <= y?=w1147:bool)
            n323 = Select(t=w1141, s=w1146, f=w1145) -> (s? t:f=w1143:fxp<+/-,48,16>)
            n324 = xnode "FPGA I/O Node"("Connector0/AO0"=w1143) -> ()  [unwired: 1 in, 1 out]
            n325 = Compound Arithmetic op=OR(w1146, w1147) -> (w1144:bool)
            n326 = call "Wait13"("Count(uSec)"=u16 100) -> ()  [unwired: 1 out]
          }
        }
        frame #7 {
          n327 = call "Wait16"("Count(uSec)"=u8 100) -> ()  [unwired: 1 out]
        }
        frame #8 {
          n328 = local write "ScanFinished?"(TRUE ("ScanFinished?")) -> ()
        }
      }
      n329 = while {
        stop <- w21 stop-if-true
        n330 = xnode ("Register Read")() -> ("Data"=w22:bool)  [unwired: 1 in, 1 out]
        n331 = xnode ("FIFO Method Node")() -> ("Number of Elements to Read"=w20:u32)  [unwired: 1 in, 1 out]
        n332 = local read "ScanFinished?"() -> (w23:bool)
        n333 = call "Wait8"("Count(uSec)"=u8 200 ("Count(mSec)")) -> ()  [unwired: 1 out]
        n334 = Or(x=w23, y=w22) -> (x .or. y?=w21:bool)
        n335 = Greater Than 0?(x=w20) -> (x > 0?=w19:bool)
        n336 = case shown="True" w19 {
          frame False {
          }
          frame True {
            # "push data in swapbuffer from target to host and clear buffer synchronously"
            n337 = flat-sequence {
              frame #0 {
              }
              frame #1 {
                n338 = xnode ("FIFO Method Node")("Timeout"=8192) -> ("Element"=w25:u8)  [unwired: 1 in, 2 out]
                n339 = case shown="2" w25 {
                  frame 0, Default {
                    n340 = flat-sequence {
                      frame #0 {
                        n341 = node-c288(refnum<k21> "8MHz" ("Source Name")) -> (w29:T1)
                        n342 = timed-loop {
                          timing: w29 -> [_]
                          timing-out: [_] -> w28
                          shift-right: [w31] -> _
                          shift-left: _ -> [w38]
                          shift-right: [w38] -> _
                          shift-left: _ -> [w37]
                          shift-right: [w37] -> _
                          shift-left: _ -> [w34]
                          tunnel: [w30] -> _
                          i -> [w30]
                          stop <- w35 stop-if-true
                          n343 = Greater Or Equal?(x=w30, y=16386) -> (x >= y?=w35:bool)
                          n344 = Greater Or Equal?(x=w30, y=3) -> (x >= y?=w33:bool)
                          n345 = case shown="True" w33 {
                            tunnel: w34 -> [_ w39]
                            frame False {
                            }
                            frame True {
                              n346 = xnode ("FIFO Method Node")("Element"=w39, "Timeout"=0) -> ()  [unwired: 1 in, 2 out]
                            }
                          }
                          n347 = xnode ("Memory Method Node")("Address"=w30) -> ("Data"=w31:fxp<+/-,48,16>)  [unwired: 1 in, 1 out]
                        }
                        n348 = node-c288(w28) -> ()
                      }
                      frame #1 {
                        n349 = node-c288() -> (w48:T1)  [unwired: 1 in]
                        n350 = timed-loop {
                          timing: w48 -> [_]
                          timing-out: [_] -> w47
                          i -> [w49]
                          stop <- w50 stop-if-true
                          n351 = xnode ("Memory Method Node")("Address"=w49, "Data"=fxp<+/-,48,16> -100.0) -> ()  [unwired: 1 in, 1 out]
                          n352 = Greater Or Equal?(x=w49, y=16383) -> (x >= y?=w50:bool)
                        }
                        n353 = node-c288(w47) -> ()
                      }
                    }
                  }
                  frame 1 {
                    n354 = flat-sequence {
                      frame #0 {
                        n355 = node-c288(refnum<k21> "8MHz" ("Source Name")) -> (w59:T1)
                        n356 = timed-loop {
                          timing: w59 -> [_]
                          timing-out: [_] -> w58
                          shift-right: [w68] -> _
                          shift-left: _ -> [w67]
                          shift-right: [w67] -> _
                          shift-left: _ -> [w66]
                          shift-right: [w66] -> _
                          shift-left: _ -> [w63]
                          i -> [w62]
                          stop <- w64 stop-if-true
                          n357 = Greater Or Equal?(x=w62, y=3) -> (x >= y?=w61:bool)
                          n358 = Greater Or Equal?(x=w62, y=16386) -> (x >= y?=w64:bool)
                          n359 = case shown="True" w61 {
                            tunnel: w63 -> [_ w69]
                            frame False {
                            }
                            frame True {
                              n360 = xnode ("FIFO Method Node")("Element"=w69, "Timeout"=0) -> ()  [unwired: 1 in, 2 out]
                            }
                          }
                          n361 = xnode ("Memory Method Node")("Address"=w62) -> ("Data"=w68:fxp<+/-,48,16>)  [unwired: 1 in, 1 out]
                        }
                        n362 = node-c288(w58) -> ()
                      }
                      frame #1 {
                        n363 = node-c288() -> (w78:T1)  [unwired: 1 in]
                        n364 = timed-loop {
                          timing: w78 -> [_]
                          timing-out: [_] -> w77
                          i -> [w79]
                          stop <- w81 stop-if-true
                          n365 = xnode ("Memory Method Node")("Address"=w79, "Data"=fxp<+/-,48,16> -100.0) -> ()  [unwired: 1 in, 1 out]
                          n366 = Greater Or Equal?(x=w79, y=16383) -> (x >= y?=w81:bool)
                        }
                        n367 = node-c288(w77) -> ()
                      }
                    }
                  }
                  frame 2 {
                    n368 = flat-sequence {
                      frame #0 {
                        n369 = node-c288(refnum<k21> "8MHz" ("Source Name")) -> (w89:T1)
                        n370 = timed-loop {
                          timing: w89 -> [_]
                          timing-out: [_] -> w88
                          shift-right: [w90] -> _
                          shift-left: _ -> [w98]
                          shift-right: [w98] -> _
                          shift-left: _ -> [w97]
                          shift-right: [w97] -> _
                          shift-left: _ -> [w94]
                          i -> [w91]
                          stop <- w95 stop-if-true
                          n371 = Greater Or Equal?(x=w91, y=3) -> (x >= y?=w93:bool)
                          n372 = Greater Or Equal?(x=w91, y=16386) -> (x >= y?=w95:bool)
                          n373 = case shown="True" w93 {
                            tunnel: w94 -> [_ w99]
                            frame False {
                            }
                            frame True {
                              n374 = xnode ("FIFO Method Node")("Element"=w99, "Timeout"=0) -> ()  [unwired: 1 in, 2 out]
                            }
                          }
                          n375 = xnode ("Memory Method Node")("Address"=w91) -> ("Data"=w90:fxp<+/-,48,16>)  [unwired: 1 in, 1 out]
                        }
                        n376 = node-c288(w88) -> ()
                      }
                      frame #1 {
                        n377 = node-c288() -> (w108:T1)  [unwired: 1 in]
                        n378 = timed-loop {
                          timing: w108 -> [_]
                          timing-out: [_] -> w107
                          i -> [w110]
                          stop <- w111 stop-if-true
                          n379 = xnode ("Memory Method Node")("Address"=w110, "Data"=fxp<+/-,48,16> -100.0) -> ()  [unwired: 1 in, 1 out]
                          n380 = Greater Or Equal?(x=w110, y=16383) -> (x >= y?=w111:bool)
                        }
                        n381 = node-c288(w107) -> ()
                      }
                    }
                  }
                }
              }
              frame #2 {
              }
            }
          }
        }
      }
    }
    frame #3 {
      n382 = local write "TargetDone?"(TRUE ("TargetDone?")) -> ()
    }
  }
